vi "Calculate Waevform.vi"(8 "Error In (no Error) In":errorcluster, 10 "Controls In":T2={"Type"=enum."Sine", "Periods"=0.0, "Points"=0, "Offset"=0.0, "Amplitdue"=0.0, "Phase"=0.0, "func"=""}, 11 "Display State In":T1={"Show Axes"=FALSE, "Show Y=0"=FALSE, "Controls"={"Type"=enum."Sine", "Periods"=0.0, "Points"=0, "Offset"=0.0, "Amplitdue"=0.0, "Phase"=0.0, "func"=""}, "Show Current Location"=FALSE, "Current Location"=0, "dt"=0.0, "t0"=timestamp(0 s since 1904-01-01), "Format and Units"="%_3p"} caption="State") -> (0 "Error Out":errorcluster, 2 "Display State Out":T1={"Show Axes"=FALSE, "Show Y=0"=FALSE, "Controls"={"Type"=enum."Sine", "Periods"=0.0, "Points"=0, "Offset"=0.0, "Amplitdue"=0.0, "Phase"=0.0, "func"=""}, "Show Current Location"=FALSE, "Current Location"=0, "dt"=0.0, "t0"=timestamp(0 s since 1904-01-01), "Format and Units"="%_3p"} caption="State", 3 "Signal Out":waveform(dbl))   [LabVIEW 2018, in "Waveform Control.xctl"]
doc: "Calculate the waveform based on the controls and update the display state"
uses:
  Waveform Control.xctl
  FP Controls.ctl
  Function Types.ctl
  Controls/Waveform State.ctl
  <vilib>/Analysis/1siggen.llb/Ramp Pattern by Samples.vi
  <vilib>/Waveform/WDTOps.llb/WDT Get Waveform Subset DBL.vi
  <vilib>/measure/NI_MABase.lvlib
  <vilib>/measure/NI_MAPro.lvlib
  <vilib>/Analysis/NI_AALBase.lvlib
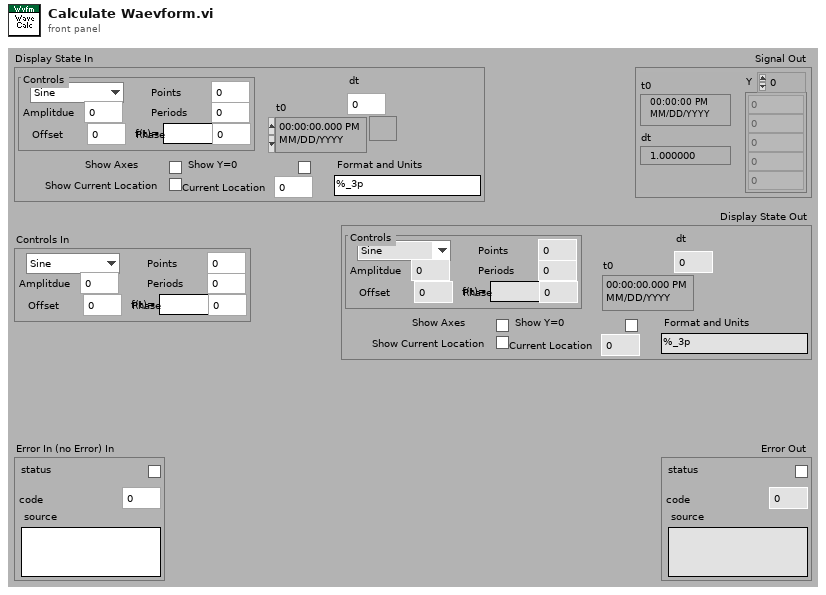
[diagram p1: front panel]
types:
  T1 = typedef "Waveform Control.xctl/Waveform State.ctl" = cluster{"Show Axes":bool, "Show Y=0":bool, "Controls":T2, "Show Current Location":bool, "Current Location":i32, "dt":dbl, "t0":timestamp, "Format and Units":string}
  T2 = typedef "Waveform Control.xctl/FP Controls.ctl" = cluster{"Type":T3, "Periods":dbl, "Points":i32, "Offset":dbl, "Amplitdue":dbl, "Phase":dbl, "func":string}
  T3 = typedef "Waveform Control.xctl/Function Types.ctl" = enum16{"Level", "Sine", "Triangle", "Ramp", "Saw Tooth", "Square", "Function"}
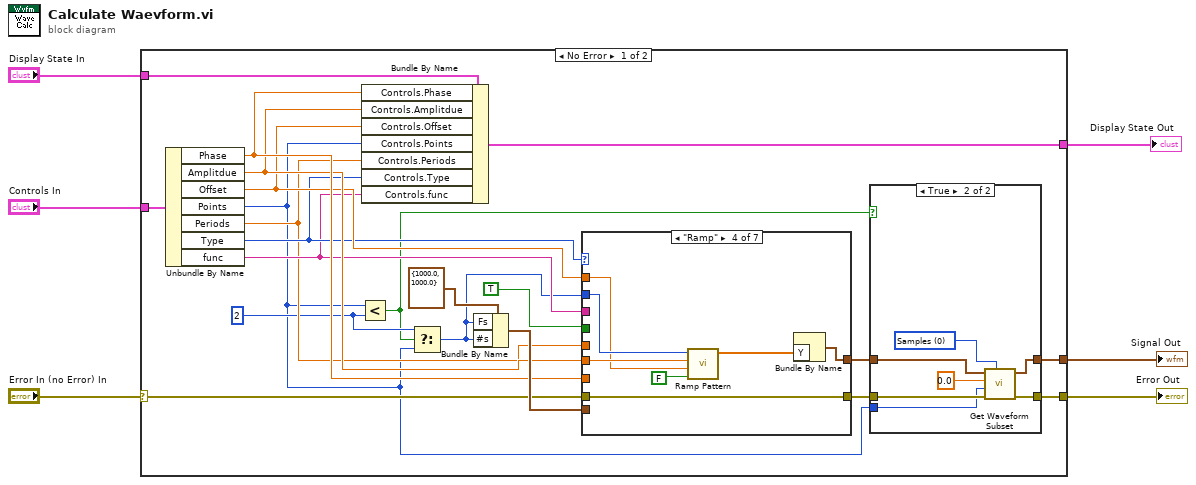
[diagram p0: block diagram]
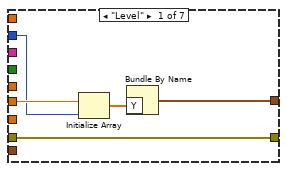
[diagram p3: hidden frame]
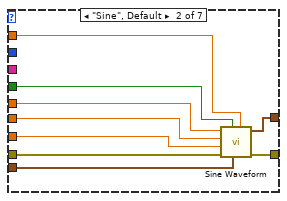
[diagram p4: hidden frame]
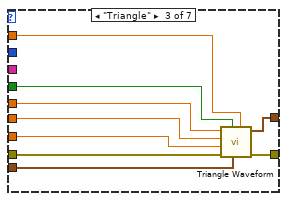
[diagram p5: hidden frame]
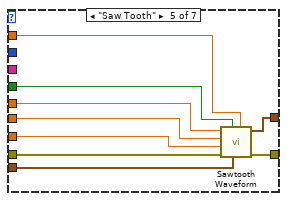
[diagram p6: hidden frame]
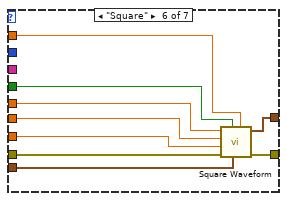
[diagram p7: hidden frame]
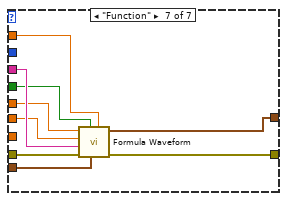
[diagram p8: hidden frame]
diagram:
  n1 = case shown="No Error" "Error In (no Error) In" {
    selector: "Error In (no Error) In" -> [w16 w95]
    tunnel: [w10 _] -> w6
    tunnel: "Controls In" -> [w27 _]
    tunnel: "Display State In" -> [w26 w94]
    tunnel: [w9 w95] -> w2
    tunnel: [w15 w94] -> w1
    frame No Error {
      w14 = 2 ("y")
      n2 = Unbundle By Name(w27) -> ("Phase"=w22:dbl, "Amplitdue"=w21:dbl, "Offset"=w20:dbl, "Points"=w8:i32, "Periods"=w17:dbl, "Type"=w19:T3, "func"=w18:string)
      n3 = Less?(x=w8, y=w14) -> (x < y?=w13:bool)
      n4 = Bundle By Name(cluster=w26, "Controls.Phase"=w22, "Controls.Amplitdue"=w21, "Controls.Offset"=w20, "Controls.Points"=w8, "Controls.Periods"=w17, "Controls.Type"=w19, "Controls.func"=w18) -> (w15:T1)
      n5 = Select(t=w14, s=w13, f=w8) -> (s? t:f=w7:i32)
      n6 = Bundle By Name(cluster=cluster{"Fs":dbl, "#s":dbl} {"Fs"=1000.0, "#s"=1000.0} ("sampling info"), "Fs"=w7, "#s"=w7) -> (w24:cluster{"Fs":dbl, "#s":dbl})
      n7 = case shown="\"Ramp\"" w19 {
        tunnel: TRUE ("reset signal") -> [_ w50 w59 _ w75 w84 w91]
        tunnel: w20 -> [_ w49 w58 w64 w74 w83 w87]
        tunnel: w21 -> [w41 w48 w57 w65 w73 w82 w89]
        tunnel: w22 -> [_ w47 w56 _ w72 w81 _]
        tunnel: w17 -> [_ w46 w55 _ w71 w80 w90]
        tunnel: w24 -> [_ w45 w54 _ w70 w79 w88]
        tunnel: [w38 w44 w53 w63 w69 w78 w92] -> w11
        tunnel: w18 -> [_ _ _ _ _ _ w93]
        tunnel: w7 -> [w40 _ _ w66 _ _ _]
        tunnel: [w37 w43 w52 w61 w68 w77 w86] -> w12
        tunnel: w16 -> [w37 w42 w51 w61 w67 w76 w85]
        frame "Level" {
          n8 = Initialize Array(w41, w40) -> (w39:dbl[])
          n9 = Bundle By Name("Y"=w39) -> (w38:waveform(dbl))  [unwired: 1 out]
        }
        frame "Sine", Default {
          n10 = call <vilib>:"Sine Waveform.vi"("offset"=w49, "sampling info"=w45, "reset signal"=w50, "error in (no error)"=w42, "phase"=w47, "amplitude"=w48, "frequency"=w46) -> ("error out"=w43:errorcluster, "signal out"=w44:waveform(dbl))  [unwired: 3 out]
        }
        frame "Triangle" {
          n11 = call <vilib>:"Triangle Waveform.vi"("offset"=w58, "sampling info"=w54, "reset signal"=w59, "error in (no error)"=w51, "phase"=w56, "amplitude"=w57, "frequency"=w55) -> ("error out"=w52:errorcluster, "signal out"=w53:waveform(dbl))  [unwired: 3 out]
        }
        frame "Ramp" {
          n12 = call-poly <vilib>:"Ramp Pattern.vi"("exclude end?"=FALSE, "start"=w64, "end"=w65, "samples"=w66) -> ("Ramp Pattern"=w62:dbl[])  [unwired: 6 in, 1 out]
          n13 = Bundle By Name("Y"=w62) -> (w63:waveform(dbl))  [unwired: 1 out]
        }
        frame "Saw Tooth" {
          n14 = call <vilib>:"Sawtooth Waveform.vi"("offset"=w74, "sampling info"=w70, "reset signal"=w75, "error in (no error)"=w67, "phase"=w72, "amplitude"=w73, "frequency"=w71) -> ("error out"=w68:errorcluster, "signal out"=w69:waveform(dbl))  [unwired: 3 out]
        }
        frame "Square" {
          n15 = call <vilib>:"Square Waveform.vi"("offset"=w83, "sampling info"=w79, "reset signal"=w84, "error in (no error)"=w76, "phase"=w81, "amplitude"=w82, "frequency"=w80) -> ("error out"=w77:errorcluster, "signal out"=w78:waveform(dbl))  [unwired: 1 in, 2 out]
        }
        frame "Function" {
          n16 = call <vilib>:"Formula Waveform.vi"("offset"=w87, "sampling info"=w88, "reset signal"=w91, "error in (no error)"=w85, "formula"=w93, "amplitude"=w89, "frequency"=w90) -> ("error out"=w86:errorcluster, "signal out"=w92:waveform(dbl))  [unwired: 3 out]
        }
      }
      n17 = case shown="True" w13 {
        tunnel: w12 -> [w28 w35]
        tunnel: w11 -> [w29 w36]
        tunnel: [w29 w33] -> w10
        tunnel: [w28 w32] -> w9
        tunnel: w8 -> [_ w30]
        frame False {
        }
        frame True {
          w31 = u16 0 items=["Samples", "Relative Time"] ("start/duration format")
          n18 = call-poly <vilib>:"Get Waveform Subset.vi"("start/duration format"=w31, "error in (no error)"=w35, "duration"=w30, "start samples/time"=0.0, "waveform in"=w36) -> ("error out"=w32:errorcluster, "waveform out"=w33:waveform(dbl))  [unwired: 3 out]
        }
      }
    }
    frame Error {
    }
  }
  "Signal Out" <- w6
  "Error Out" <- w2
  "Display State Out" <- w1
